vi "Write USB Port.vi"(8 "error in (no error)":errorcluster, 10 "camera session":T1, 11 "USB Camera in":refnum<class "USB Camera.lvclass">) -> (0 "error out":errorcluster, 3 "USB Camera out":refnum<class "USB Camera.lvclass">)   [LabVIEW 2020, in "USB Camera.lvclass"]
uses:
  USB Camera.lvclass
  <vilib>/userdefined/High Color/IMAQdx.ctl
  USB Camera.lvclass/USB Camera.ctl
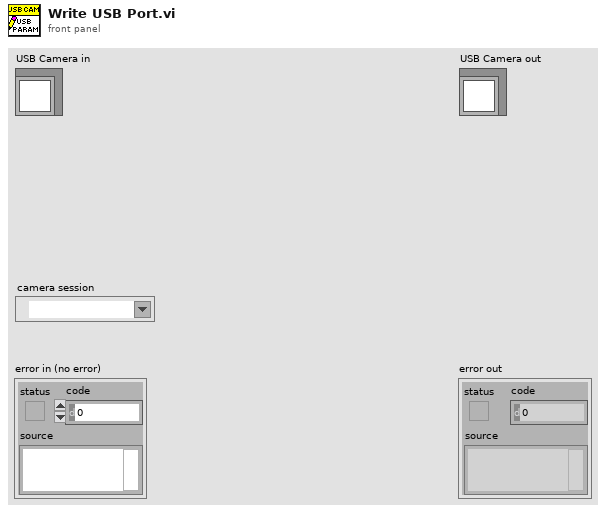
[diagram p1: front panel]
types:
  T1 = typedef "IMAQdx.ctl" = refnum<k21>
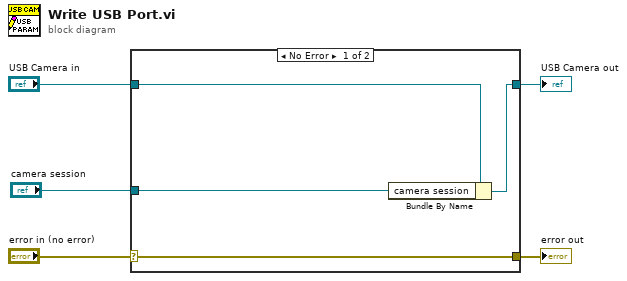
[diagram p0: block diagram]
diagram:
  n1 = case shown="No Error" "error in (no error)" {
    selector: "error in (no error)" -> [w9 w10]
    tunnel: [w9 w10] -> w4
    tunnel: [w7 w11] -> w2
    tunnel: "USB Camera in" -> [w8 w11]
    tunnel: "camera session" -> [w6 _]
    frame No Error {
      n2 = Bundle By Name(cluster=w8, "camera session"=w6) -> (w7:refnum<class "USB Camera.lvclass">)
    }
    frame Error {
    }
  }
  "error out" <- w4
  "USB Camera out" <- w2
